vi "ADC Checker.vi"(0 "Pump Data":T2={"Voltages"=[0.015201568603515625, 0.00335693359375, 0.003021240234375, 0.12260055541992188, 0.06085968017578125, 0.052234649658203125], "PumpCurrent"=[0.015201568603515625, 0.00335693359375, 0.003021240234375, 0.12260055541992188, 0.06085968017578125, 0.052234649658203125], "Speed"=[0.0, 0.0, 0.0, 0.0, 0.0, 0.0], "ControllerCurrent"=[0.015201568603515625, 0.00335693359375, 0.003021240234375, 0.12260055541992188, 0.06085968017578125, 0.052234649658203125], "Pressure"=[0.015201568603515625, 0.00335693359375, 0.003021240234375, 0.12260055541992188, 0.06085968017578125, 0.052234649658203125], "Flow"=[0.0, 0.0, 0.0, 0.125, 0.0625, 0.0625], "Elapsed Time (Display)"=[7.1, 7.1, 7.1, 458133.45, 458138.85000000003, 458126.75], "Avg Pressure"=0.0, "Avg Speed"=0.0, "Elapsed Time"=[4074.9003000000002, 4074.9003000000002, 4074.9003000000002, 4074.9003000000002, 4074.9003000000002, 4074.9003000000002]} {"Elapsed Time" format="%<%H:%M:%S>t"; "Elapsed Time (Display)" format="%<%H:%M:%S>t"; "Speed" format="%#_4f"; "ControllerCurrent" format="%#.1g"; "Pressure" format="%#.0f"; "Flow" format="%#.0f"; "PumpCurrent" format="%#.1g"; "Voltages" format="%#.0f"}, 5 "Run Profile":bool, 7 "Pumps Present":bool[](array[boolean]), 9 "Not Stopped":bool[](array[boolean])) -> (4 "Reset ADCs":bool)   [LabVIEW 2019]
uses:
  Controls/Pump Data.ctl
panel:
  in  "Enable":bool=TRUE
  out "snapshot array":T1(array[cluster])
  out "output array":T1(array[cluster])
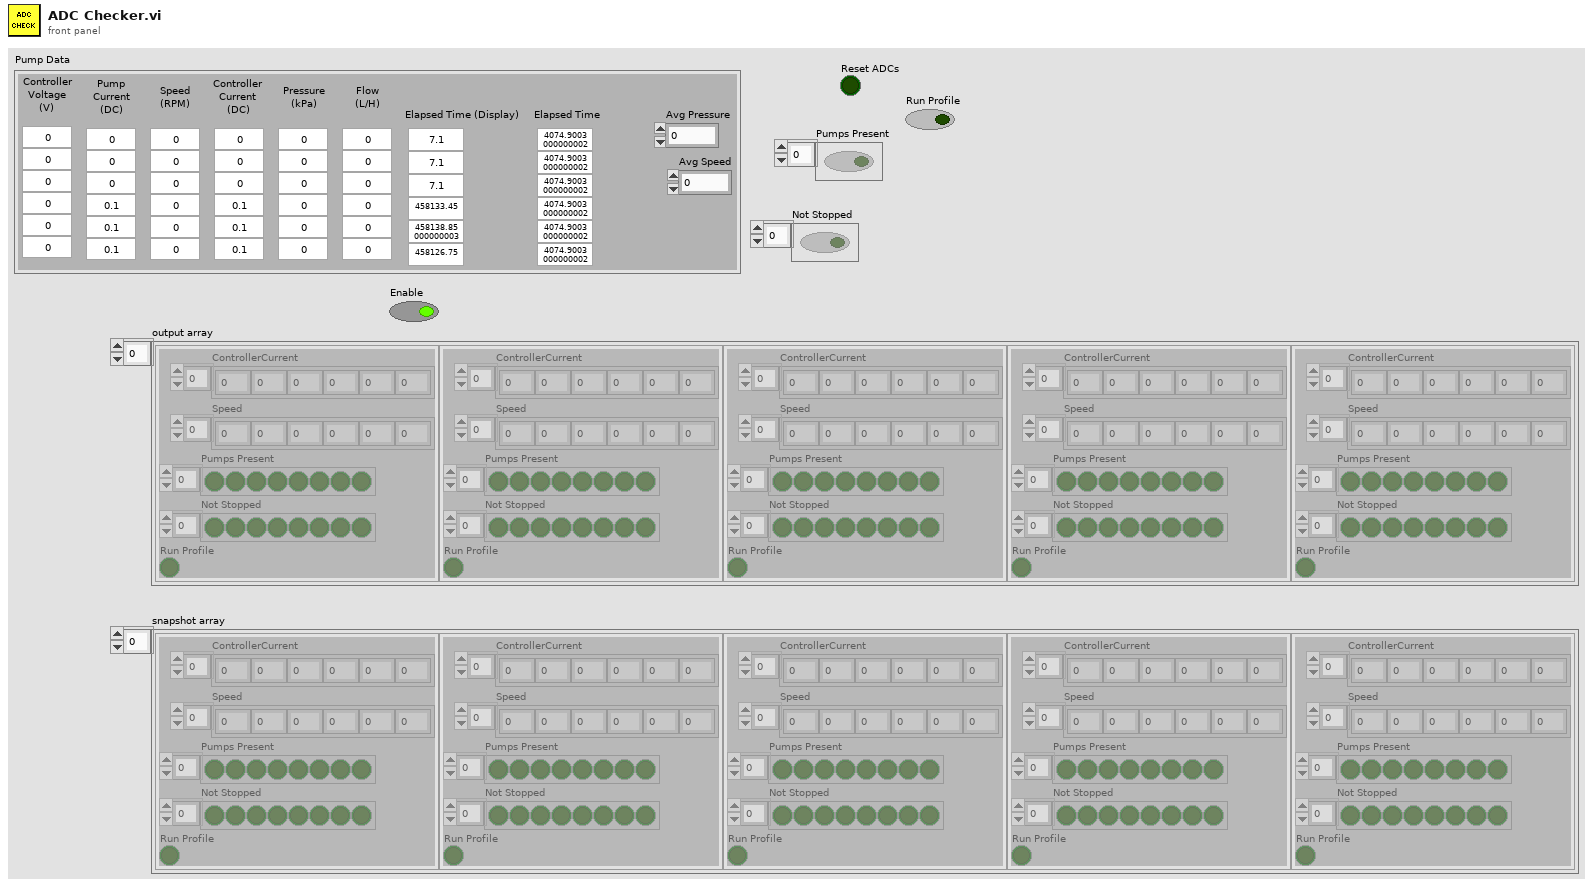
[diagram p1: front panel]
types:
  T1 = cluster{"ControllerCurrent":dbl[], "Speed":dbl[], "Pumps Present":bool[], "Not Stopped":bool[], "Run Profile":bool}[]
  T2 = typedef "Pump Data.ctl" = cluster{"Voltages":dbl[], "PumpCurrent":dbl[], "Speed":dbl[], "ControllerCurrent":dbl[], "Pressure":dbl[], "Flow":dbl[], "Elapsed Time (Display)":dbl[], "Avg Pressure":dbl, "Avg Speed":dbl, "Elapsed Time":dbl[]}
  T3 = cluster{"ControllerCurrent":dbl[], "Speed":dbl[], "Pumps Present":bool[], "Not Stopped":bool[], "Run Profile":bool}
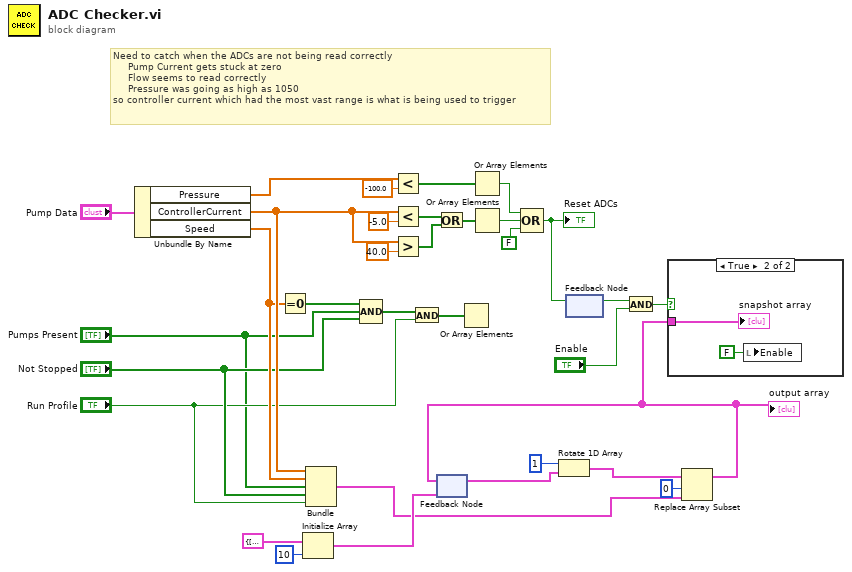
[diagram p0: block diagram]
diagram:
  # "Need to catch when the ADCs are not being read correctly\n     Pump Current gets stuck at zero\n     Flow seems to read correctly\n     Pressure was going as high as 1050\nso controller current which had the most vast range is what is being used to trigger"
  n1 = Unbundle By Name("Pump Data") -> ("Pressure"=w9:dbl[], "ControllerCurrent"=w25:dbl[], "Speed"=w24:dbl[])
  n2 = Equal To 0?(x=w24) -> (x = 0?=w2:bool[])
  n3 = Initialize Array(T3 {"ControllerCurrent"=[], "Speed"=[], "Pumps Present"=[], "Not Stopped"=[], "Run Profile"=FALSE} ("output cluster"), 10 ("dimension size")) -> (w19:T1)
  n4 = Bundle("ControllerCurrent"=w25, "Speed"=w24, "Pumps Present"="Pumps Present", "Not Stopped"="Not Stopped", "Run Profile"="Run Profile") -> (w15:T3)  [unwired: 1 in]
  n5 = Compound Arithmetic op=AND(w2, "Pumps Present", "Not Stopped") -> (w27:bool[])
  n6 = Less?(x=w9, y=-100.0) -> (x < y?=w6:bool[])
  n7 = Less?(x=w25, y=-5.0) -> (x < y?=w32:bool[])
  n8 = Greater?(x=w25, y=40.0) -> (0:w31:bool[])
  n9 = And(x=w27, y="Run Profile") -> (x .and. y?=w26:bool[])
  n10 = Or(x=w32, y=w31) -> (x .or. y?=w28:bool[])
  n11 = feedback #1(w19) -> (w18:T1)
  n12 = Or Array Elements(Boolean array=w26) -> ()  [unwired: 1 out]
  n13 = Or Array Elements(Boolean array=w6) -> (logical OR=w5:bool)
  n14 = Or Array Elements(Boolean array=w28) -> (logical OR=w7:bool)
  n15 = Compound Arithmetic op=OR(w5, w7, FALSE ("value")) -> (w4:bool)
  "Reset ADCs" <- w4
  n16 = Rotate 1D Array(1:w18, 2:1 ("n")) -> (0:w16:T1)
  n17 = feedback-in #2(w4) -> ()
  n18 = feedback #2() -> (w13:bool)  [unwired: 1 in]
  n19 = And(x=w13, y="Enable") -> (x .and. y?=w11:bool)
  n20 = Replace Array Subset(array=w16, new element=w15, index=0) -> (w10:T1)
  "output array" <- w10
  n21 = feedback-in #1(w10) -> ()
  n22 = case shown="True" w11 {
    tunnel: w10 -> [_ w35]
    frame False {
    }
    frame True {
      n23 = local write "Enable"(FALSE ("Enable")) -> ()
      "snapshot array" <- w35
    }
  }
